vi "FGVInaSingleCode.vi"() -> ()   [LabVIEW 2019]
panel:
  out "Data Output 2":dbl
  out "Data Output":dbl
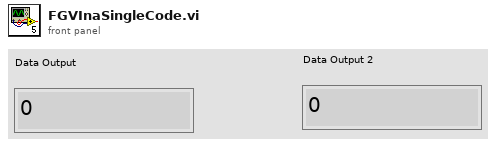
[diagram p1: front panel]
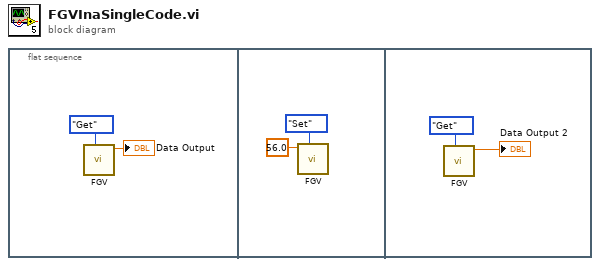
[diagram p0: block diagram]
diagram:
  n1 = flat-sequence {
    frame #0 {
      n2 = call "FGV.vi"("State"=enum16{"Set", "Get"}."Get") -> ("Data Output"=→"Data Output":dbl)  [unwired: 10 in]
    }
    frame #1 {
      n3 = call "FGV.vi"("State"=enum16{"Set", "Get"}."Set", "Data Input"=56.0) -> ()  [unwired: 9 in, 1 out]
    }
    frame #2 {
      n4 = call "FGV.vi"("State"=enum16{"Set", "Get"}."Get") -> ("Data Output"=→"Data Output 2":dbl)  [unwired: 10 in]
    }
  }
